vi "hse-application_SetApplicationUnitID.vi"(8 "error in":errorcluster, 10 "Unit-ID":string) -> (0 "error out":errorcluster)   [LabVIEW 2020, in "hse-application.lvclass"]
doc: "Manually set the application \"Unit ID\".\n\n____\nHAMPEL SOFTWARE ENGINEERING v3.8.0 (2023-12-18 14:41)"
uses:
  hse-application.lvclass
  hse-misc/Controls/FGV_Actions.ctl
  hse-misc/hse-misc.lvlib
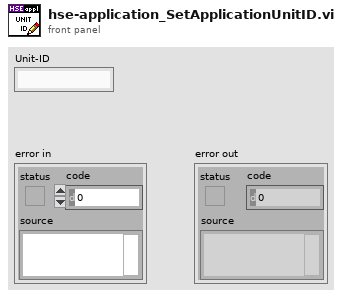
[diagram p1: front panel]
types:
  T1 = typedef "hse-misc.lvlib/FGV_Actions.ctl" = enum16{"Set", "Get"}
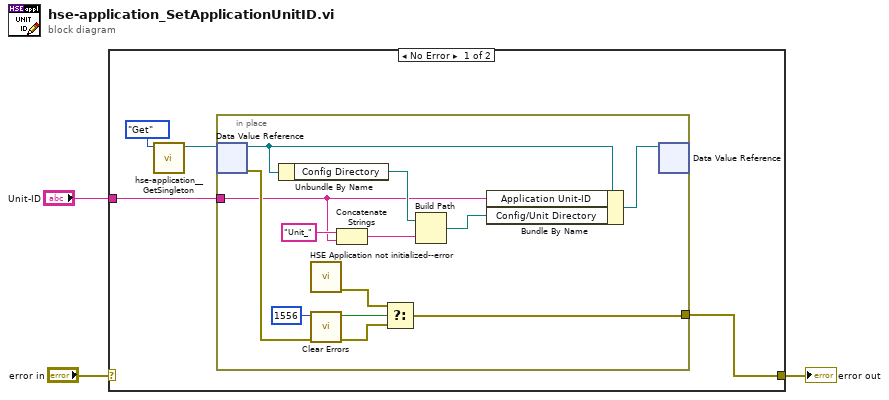
[diagram p0: block diagram]
diagram:
  n1 = case shown="No Error" "error in" {
    selector: "error in" -> [_ w21]
    tunnel: [w7 w21] -> w2
    tunnel: "Unit-ID" -> [w6 _]
    frame No Error {
      n2 = call "hse-application__GetSingleton.vi"("Action"=FGV_Actions."Get") -> ("ApplicationClass DVR"=w4:refnum<data-value>)  [unwired: 9 in, 1 out]
      n3 = in-place "In Place Element Structure" {
        in-place-border: w6 -> [w13]
        in-place-border: [w17] -> w7
        n4 = in-place-dvr #1(w4) -> (w11:refnum<class "hse-application.lvclass">, w18:errorcluster)
        n5 = Unbundle By Name(w11) -> ("Config Directory"=w15:path)
        n6 = call "HSE Application not initialized--error.vi"() -> ("error out"=w20:errorcluster)  [unwired: 11 in]
        n7 = call <vilib>:"Clear Errors.vi"("error in (no error)"=w18, "specific error code to clear (0: all)"=1556) -> ("error out"=w19:errorcluster, "specific error cleared?"=w8:bool)  [unwired: 4 in]
        n8 = Concatenate Strings("Unit_" ("name or relative path"), w13) -> (w14:string)
        n9 = Select(t=w20, s=w8, f=w19) -> (s? t:f=w17:errorcluster)
        n10 = Build Path(base path=w15, name or relative path=w14) -> (appended path=w12:path)
        n11 = Bundle By Name(cluster=w11, "Application Unit-ID"=w13, "Config/Unit Directory"=w12) -> (w10:refnum<class "hse-application.lvclass">)
        n12 = in-place-dvr #1(w10) -> ()  [unwired: 2 out]
      }
    }
    frame Error {
    }
  }
  "error out" <- w2
